vi "ROI entry-Previous ROI compat-Frame size.vi"(8 "error in (no error)":errorcluster, 9 "Proceed":bool=TRUE, 11 "Old ROI file path":path) -> (0 "error out":errorcluster, 1 "Proceed":bool, 2 "ROI fit info":T1 {"ROI fit info"."Frame size"."Old" items=["100X100"=100, "128X128"=128, "200X200"=200, "256X256"=256, "512X512"=512, "1024x1024"=1024, "2048x2048"=2048]; "ROI fit info"."Frame size"."New" items=["100X100"=100, "128X128"=128, "200X200"=200, "256X256"=256, "512X512"=512, "1024x1024"=1024, "2048x2048"=2048]}, 3 "Old ROI file path (dup)":path)   [LabVIEW 2020]
uses:
  Typedefs/ROI fitting info cluster.ctl
  Typedefs/Frame Size.ctl
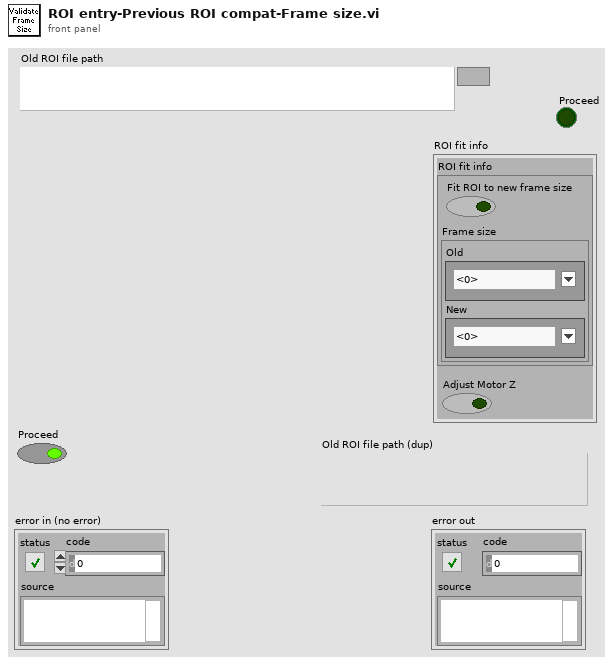
[diagram p1: front panel]
types:
  T1 = typedef "ROI fitting info cluster.ctl" = cluster{"ROI fit info":cluster{"Fit ROI to new frame size":bool, "Frame size":cluster{"Old":T2, "New":T2}}, "Adjust Motor Z":bool}
  T2 = typedef "Frame Size.ctl" = u16
  T3 = typedef "Fixed strings.ctl" = cluster{"ROI file name":string, "Normalised ROI file name":string, "Zplane Pockels values file name":string, "Functional data folder name":string, "Experiment Header file name":string, "Z-stack images folder name":string, "Groups setup rel. path":string, "Groups text file rel. path":string, "TDMS files folder name (F.img)":string, "TDMS files folder name (V.acq)":string, "TDMS files folder name (Pl.acq)":string, "Cycle rel times sequence file":string, "Dynamically called VIs folder name":string, "Time Series folder base name":string}
  T4 = typedef "AOL_Globals.ctl" = cluster{"Imaging Protocol":T5, "Number of POI":u16, "Number of Miniscans":u16, "Number of Trials":u16, "Number of Cycles ":u64, "# Averaged Frames":u16, "Laser power (%)":u8, "Pockels (V)":dbl, "Acquisition Length (sec)":dbl, "Fill time (us)":dbl, "POI Dwell time (us)":dbl, "Miniscan Dwell time per pixel (us)":dbl, "PMT 1":dbl, "PMT 2":dbl, "Back Apperture (mA)":dbl, "Frame Size":T2, "Center Frequency":dbl, "Field of View (norm)":dbl, "DwellTime (us)":dbl, "Wavelength (nm)":dbl, "Zoom":dbl, "AOL Z":dbl, "AOL Mode":T6, "GridXY":dbl, "GridZ":dbl, "TriggerPeriod (sec)":dbl, "Number of Pixels in Miniscan":u16, "Experiment folder path":path, "X centre":dbl, "Y centre":dbl, "Angle (degrees)":dbl, "Plane Mode":T7, "Threshold":u16[], "Regenerate Chirps":bool, "Rectangle ROI length (pixels)":u16, "Rectangle ROI height (pixels)":u16, "AOD fill":u16, "StartupDelay":i32, "Samples Wait after Trigger":u16, "Slip Cycle":u32, "Add Cycle":bool, "Functional Mode":T8, "Z Start":dbl, "Z Stop":dbl, "# Planes":i32, "Total Pixels":i32, "Variable Miniscan Pixels":u16[], "Use Variable Length":bool, "Use Variable Resolution":bool, "Laser power (%) at Z Start":u8, "Laser power (%) at Z Stop":u8, "Ref Z Step":i8, "Ref Dwell Time (us)":dbl, "Field of View (um)":dbl}
  T5 = typedef "Imaging Protocols enum.ctl" = enum16{"AOL Z-Stack", "Motor Z Stack", "Functional Acquisition", "Single Plane Acquisition", "Volume Acquisition", "Live Imaging", "Live Plane Imaging", "Live Volume Imaging"}
  T6 = typedef "AOL modes.ctl" = enum16{"Raster", "Structural", "Pointing", "Mini Scan", "Alignment"}
  T7 = typedef "Plane Mode.ctl" = u16
  T8 = typedef "Functional Mode.ctl" = enum16{"Point", "Line", "Patch", "Plane", "Volume"}
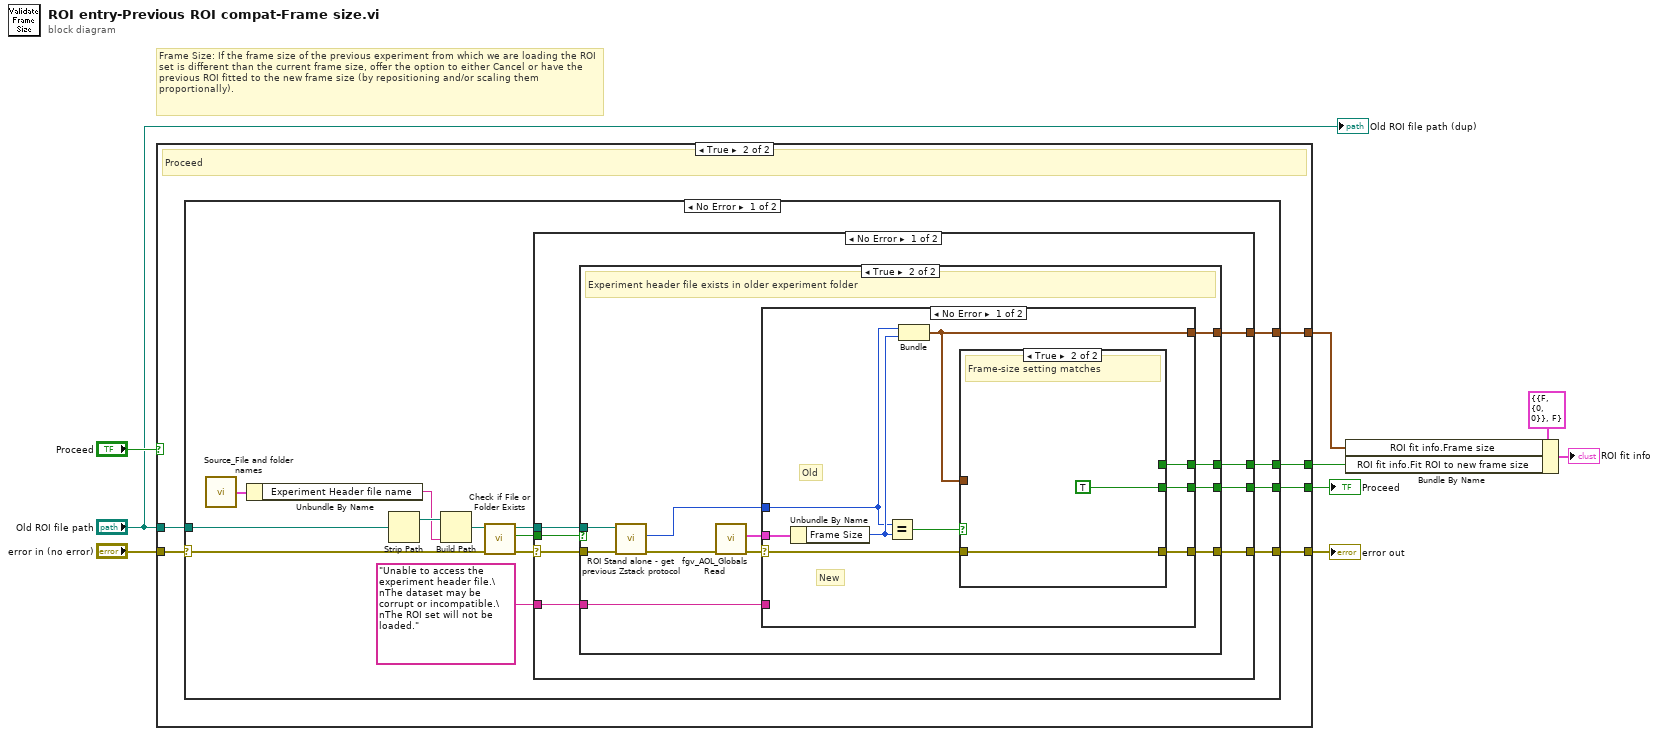
[diagram p0: block diagram]
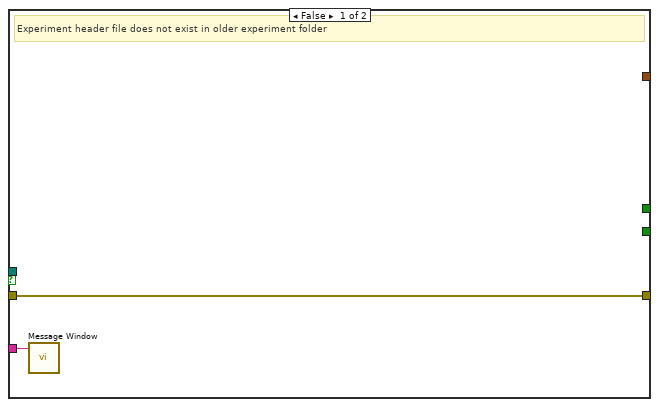
[diagram p3: hidden frame]
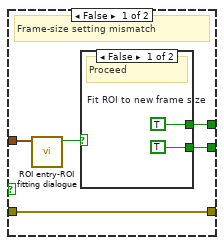
[diagram p4: hidden frame]
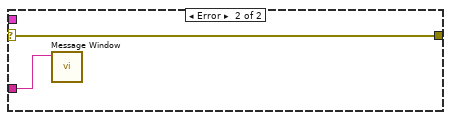
[diagram p6: hidden frame]
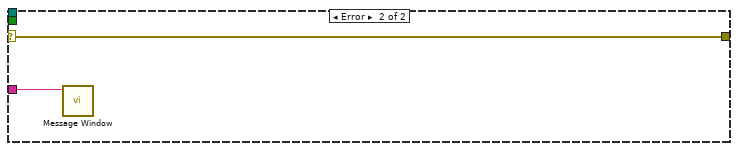
[diagram p7: hidden frame]
diagram:
  # "Frame Size: If the frame size of the previous experiment from which we are loading the ROI set is different than the current frame size, offer the option to either Cancel or have the previous ROI fitted to the new frame size (by repositioning and/or scaling them proportionally)."
  n1 = case shown="True" "Proceed" {
    tunnel: "Old ROI file path" -> [_ w16]
    tunnel: [w10 w15] -> w9
    tunnel: "error in (no error)" -> [w10 w14]
    tunnel: [_ w13] -> w7
    tunnel: [_ w12] -> w4
    tunnel: [_ w11] -> w1
    frame False {
      # "Skip"
    }
    frame True {
      # "Proceed"
      n2 = case shown="No Error" w14 {
        selector: w14 -> [w21 w74]
        tunnel: w16 -> [w28 _]
        tunnel: [w24 _] -> w13
        tunnel: [w20 w74] -> w15
        tunnel: [w18 _] -> w12
        tunnel: [w17 _] -> w11
        frame No Error {
          n3 = call "Source_File and folder names.vi"() -> ("Fixed strings"=w29:T3)  [unwired: 1 in]
          n4 = Unbundle By Name(w29) -> ("Experiment Header file name"=w26:string)
          n5 = Strip Path(path=w28) -> (stripped path=w27:path)  [unwired: 1 out]
          n6 = Build Path(base path=w27, name or relative path=w26) -> (appended path=w30:path)
          n7 = call <vilib>:"Check if File or Folder Exists.vi"("error in (no error)"=w21, "path"=w30) -> ("error out"=w22:errorcluster, "file or folder exists?"=w25:bool, "dup path"=w23:path)  [unwired: 7 in]
          n8 = case shown="No Error" w22 {
            selector: w22 -> [w35 w73]
            tunnel: w25 -> [w38 _]
            tunnel: [w37 _] -> w24
            tunnel: w23 -> [w36 _]
            tunnel: [w34 w73] -> w20
            tunnel: "Unable to access the experiment header file.\nThe dataset may be corrupt or incompatible.\nThe ROI set will not be loaded." ("Message string") -> [w33 w72]
            tunnel: [w32 _] -> w18
            tunnel: [w31 _] -> w17
            frame No Error {
              n9 = case shown="True" w38 {
                tunnel: [_ w50] -> w37
                tunnel: w36 -> [_ w43]
                tunnel: w35 -> [w40 w44]
                tunnel: [w40 w49] -> w34
                tunnel: w33 -> [w39 w47]
                tunnel: [_ w46] -> w32
                tunnel: [_ w45] -> w31
                frame False {
                  # "Experiment header file does not exist in older experiment folder"
                  n10 = call "Message Window.vi"("Message string"=w39) -> ()  [unwired: 10 in, 1 out]
                }
                frame True {
                  # "Experiment header file exists in older experiment folder"
                  n11 = call "ROI Stand alone - get previous Zstack protocol.vi"("error in (no error)"=w44, "path"=w43) -> ("error out"=w42:errorcluster, "Frame Size"=w41:T2)  [unwired: 5 in, 3 out]
                  n12 = call "fgv_AOL_Globals Read.vi"("error in (no error)"=w42) -> ("error out"=w48:errorcluster, "AOL_Globals"=w51:T4)  [unwired: 8 in, 1 out]
                  n13 = case shown="No Error" w48 {
                    selector: w48 -> [w58 w71]
                    tunnel: w51 -> [w57 _]
                    tunnel: [w60 _] -> w50
                    tunnel: [w59 w71] -> w49
                    tunnel: w47 -> [_ w70]
                    tunnel: [w56 _] -> w46
                    tunnel: [w54 _] -> w45
                    tunnel: w41 -> [w52 _]
                    frame No Error {
                      # "New"
                      # "Old"
                      n14 = Unbundle By Name(w57) -> ("Frame Size"=w55:T2)
                      n15 = Equal?(x=w52, y=w55) -> (x = y?=w53:bool)
                      n16 = Bundle("Frame Size"=w52, "Frame Size"=w55) -> (w54:cluster{"Frame Size":T2, "Frame Size":T2})  [unwired: 1 in]
                      n17 = case shown="True" w53 {
                        tunnel: [w64 TRUE] -> w60
                        tunnel: w58 -> [w63 w68]
                        tunnel: [w63 w68] -> w59
                        tunnel: [w62 _] -> w56
                        tunnel: w54 -> [w61 _]
                        frame False {
                          # "Frame-size setting mismatch"
                          n18 = call "ROI entry-ROI fitting dialogue.vi"("Frame size"=w61) -> ("Cancelled (Left button pressed)"=w65:bool)  [unwired: 10 in]
                          n19 = case shown="False" w65 {
                            tunnel: [TRUE _] -> w64
                            tunnel: [w66 _] -> w62
                            frame False {
                              w66 = TRUE  # Fit ROI to new frame size
                              # "Proceed"
                            }
                            frame True {
                              # "Cancelled"
                            }
                          }
                        }
                        frame True {
                          # "Frame-size setting matches"
                        }
                      }
                    }
                    frame Error {
                      n20 = call "Message Window.vi"("Message string"=w70) -> ()  [unwired: 10 in, 1 out]
                    }
                  }
                }
              }
            }
            frame Error {
              n21 = call "Message Window.vi"("Message string"=w72) -> ()  [unwired: 10 in, 1 out]
            }
          }
        }
        frame Error {
        }
      }
    }
  }
  "error out" <- w9
  "Proceed" <- w7
  n22 = Bundle By Name(cluster=T1 {"ROI fit info"={"Fit ROI to new frame size"=FALSE, "Frame size"={"Old"=0, "New"=0}}, "Adjust Motor Z"=FALSE} ("ROI fit info"), "ROI fit info.Frame size"=w1, "ROI fit info.Fit ROI to new frame size"=w4) -> (→"ROI fit info":T1)
  "Old ROI file path (dup)" <- "Old ROI file path"
